vi "Sub_serial_Read_byte_until_0D0A.vi"(8 "에러 입력(에러 없음)":errorcluster, 11 "VISA 참조 번호 입력":refnum<visa-resource-name>) -> (0 "에러 출력":errorcluster, 2 "버퍼 읽기":string, 3 "VISA 참조 번호 출력":refnum<visa-resource-name>)   [LabVIEW 2015]
panel:
  in  "Timeout(1sec)":dbl=1.0
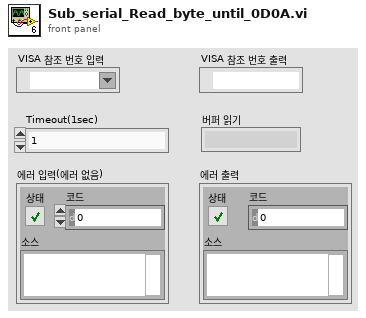
[diagram p1: front panel]
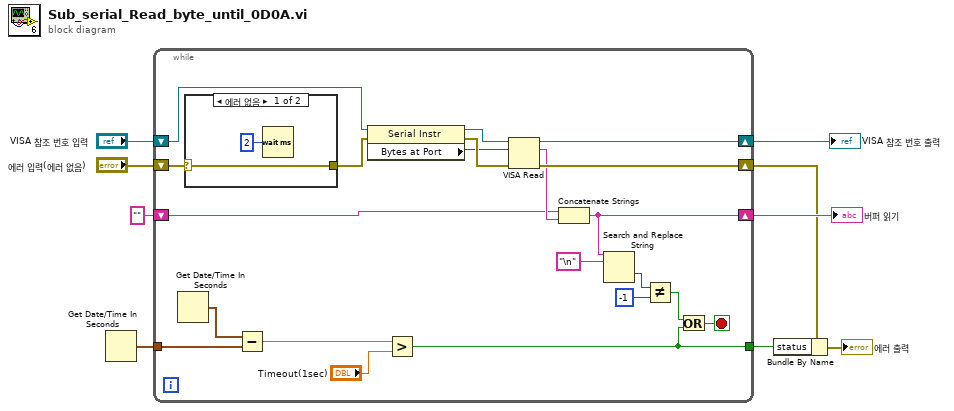
[diagram p0: block diagram]
diagram:
  n1 = Get Date/Time In Seconds() -> (seconds since 1Jan1904=w5:timestamp)
  n2 = while {
    shift-right: [w25] -> w7
    shift-left: "VISA 참조 번호 입력" -> [w30]
    shift-right: [w26] -> w3
    shift-left: "에러 입력(에러 없음)" -> [w28]
    shift-right: [w20] -> w4
    shift-left: "" -> [w21]
    tunnel: w5 -> [w16]
    tunnel: [w10] -> w2
    stop <- w12 stop-if-true
    n3 = Get Date/Time In Seconds() -> (seconds since 1Jan1904=w15:timestamp)
    n4 = case shown="에러 없음" w28 {
      selector: w28 -> [w32 w33]
      tunnel: [w32 w33] -> w29
      frame No Error {
        n5 = Wait (ms)(milliseconds to wait=u32 2 ("대기 시간(ms)")) -> ()  [unwired: 1 out]
      }
      frame Error {
      }
    }
    n6 = Subtract(x=w15, y=w16) -> (x-y=w13:dbl)
    n7 = property class="Serial Instr"(reference=w30, error in=w29) -> (reference out=w24:refnum<visa-resource-name>, error out=w27:errorcluster, "Bytes at Port"=w23:u32)
    n8 = Greater?(x=w13, y="Timeout(1sec)") -> (0:w10:bool)
    n9 = VISA Read(VISA resource name=w24, byte count=w23, error in (no error)=w27) -> (VISA resource name out=w25:refnum<visa-resource-name>, read buffer=w22:string, error out=w26:errorcluster)  [unwired: 1 out]
    n10 = Concatenate Strings(w21, w22) -> (w20:string)
    n11 = Search and Replace String(input string=w20, search string="\n") -> (offset past replacement=w18:i32)  [unwired: 6 in, 3 out]
    n12 = Not Equal?(x=w18, y=-1) -> (x != y?=w11:bool)
    n13 = Or(x=w11, y=w10) -> (x .or. y?=w12:bool)
  }
  "VISA 참조 번호 출력" <- w7
  "버퍼 읽기" <- w4
  n14 = Bundle By Name(cluster=w3, "status"=w2) -> (→"에러 출력":errorcluster)
